vi "UI Tubing Install.vi"(8 "error in":errorcluster) -> (0 "error out":errorcluster)   [LabVIEW 2019, in "Test.lvlib"]
uses:
  Test.lvlib
  Fluidic Process/SubVI/Fluidic Para.ctl
  <vilib>/Utility/file.llb/Read Delimited Spreadsheet (string).vi
  Controller/Controller.lvlib
  Queues/Queues.lvlib
  Fluidic Process/Fluidic Process.lvlib
panel:
  out "Tubing Install":bool
  in  "Stop Process":bool
  out "Remaining Time(s)":dbl
  out "Total Process":string
  out "Current Process":string
  out "Gauge":dbl(knob)=1.2869315802184793e-48 scale=0.0..100.0
  in  "Tubing Install":bool
  in  "Back":bool
  # "/"
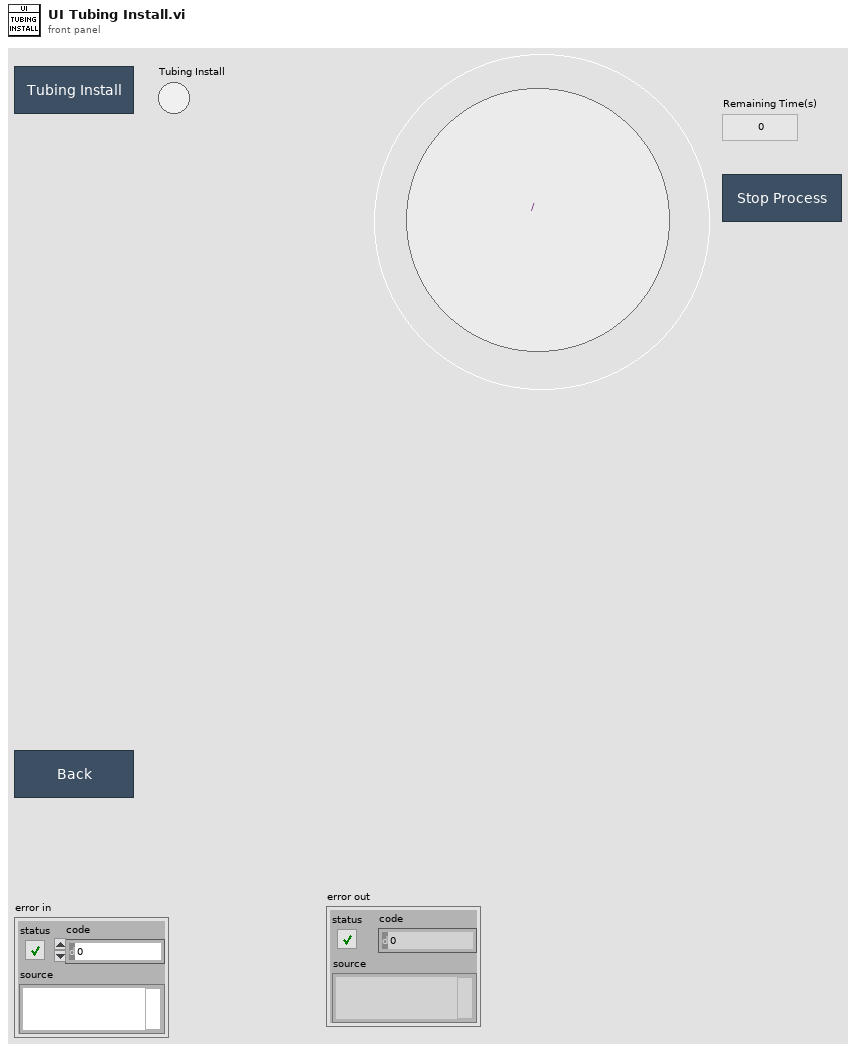
[diagram p1: front panel]
types:
  T1 = enum8{"Enabled", "Disabled", "Disabled and Grayed Out"}
  T2 = typedef "Fluidic Process.lvlib/Fluidic Para.ctl" = cluster{"Read Force Sensor":i32, "Read Regulator":i32, "Read Force Sensor?":bool, "Read Regulator?":bool, "Read Syringe Pump":i32, "Read Syringe Pump?":bool}
  T3 = typedef "Fluidic Process.lvlib/SEQ Data.ctl" = cluster{"Fluidic Process Done?":bool, "Current Process":i32, "Remaining Time":dbl, "Total Process":i32, "Air Sealing":bool, "Force Condition":bool}
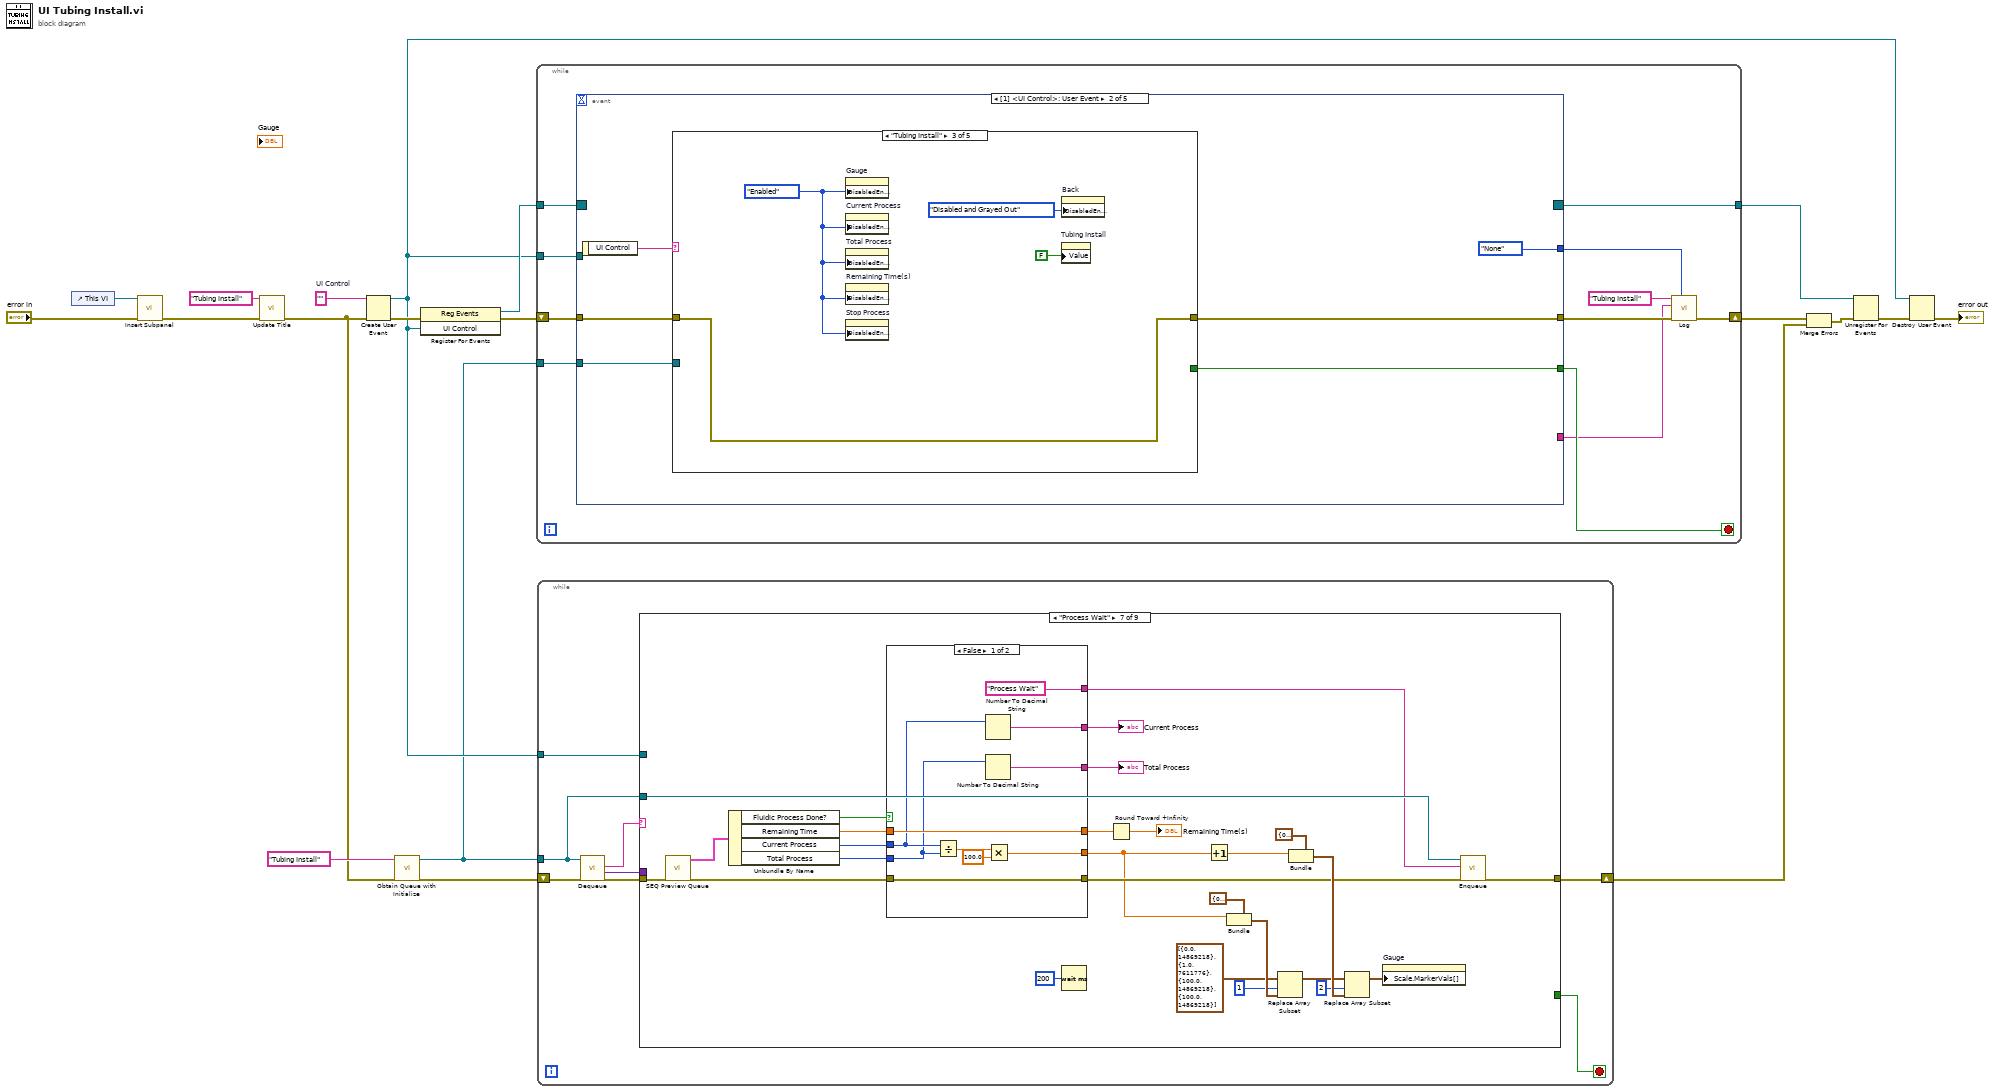
[diagram p0: block diagram]
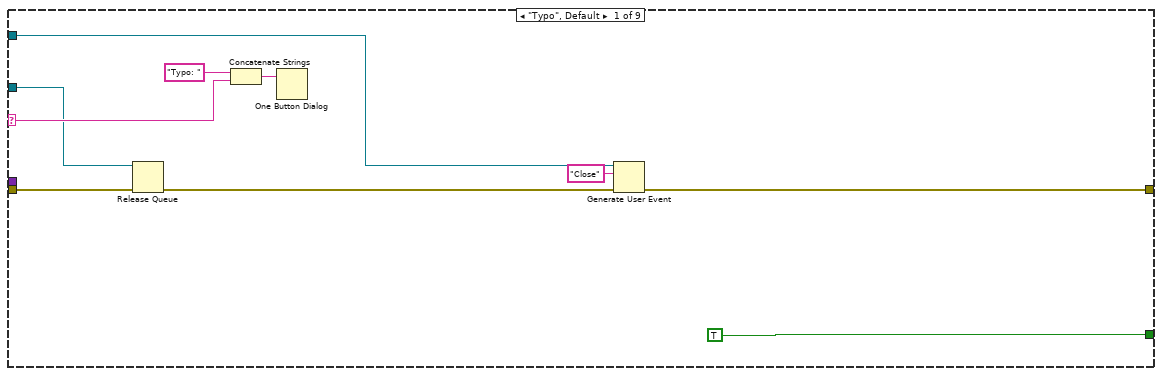
[diagram p2: hidden frame]
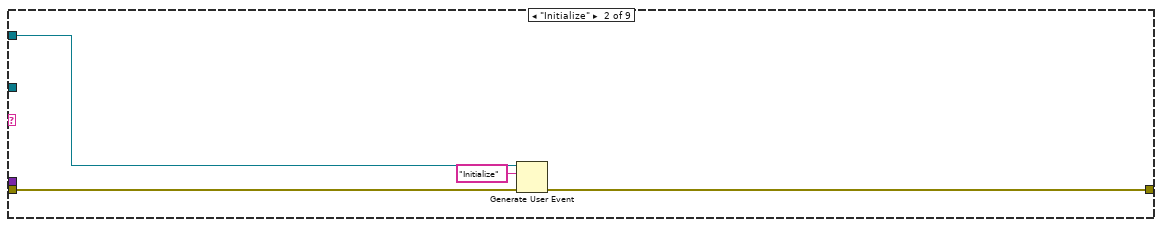
[diagram p3: hidden frame]
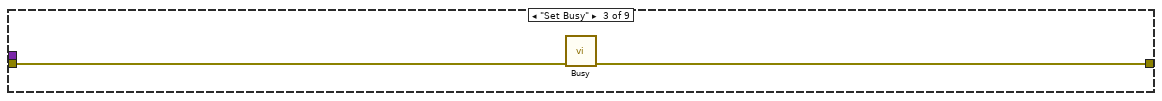
[diagram p4: hidden frame]
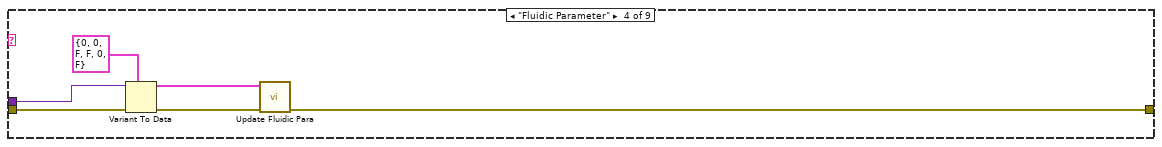
[diagram p5: hidden frame]
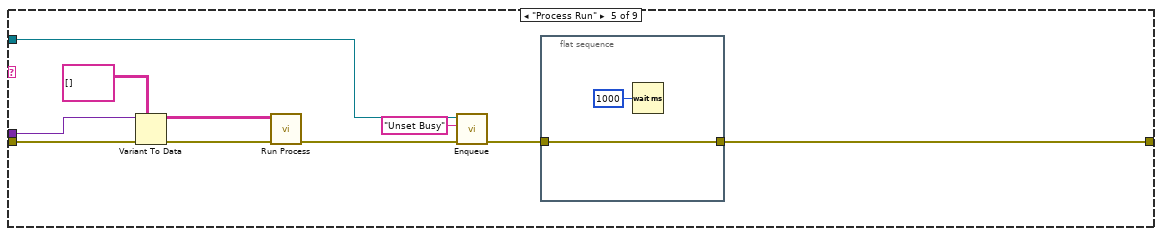
[diagram p6: hidden frame]
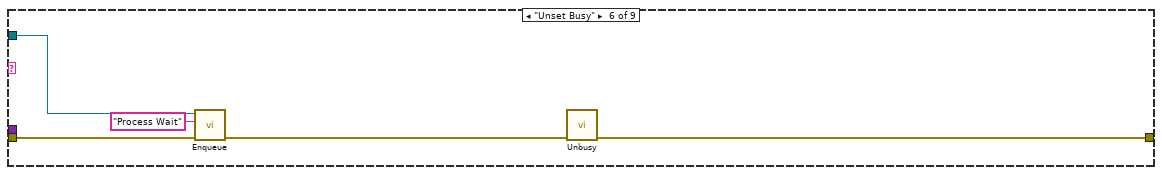
[diagram p7: hidden frame]
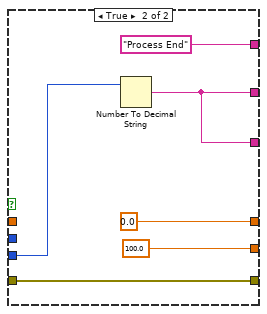
[diagram p8: hidden frame]
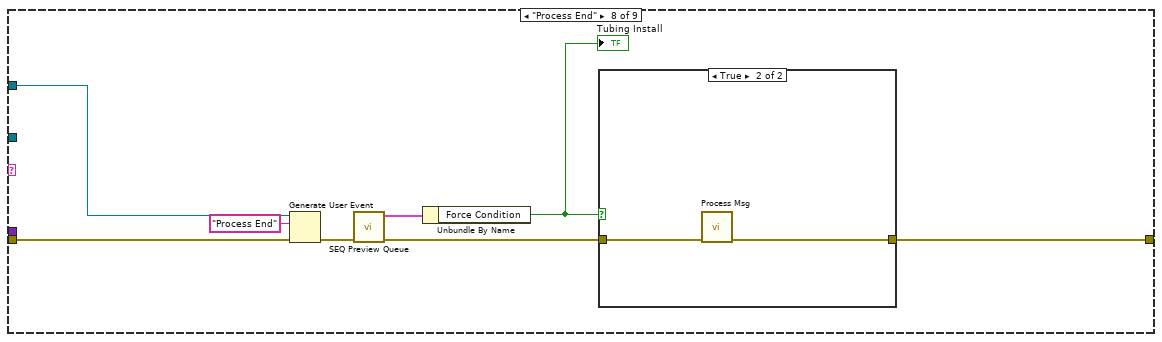
[diagram p9: hidden frame]
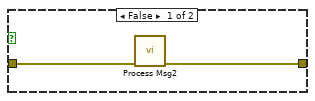
[diagram p10: hidden frame]
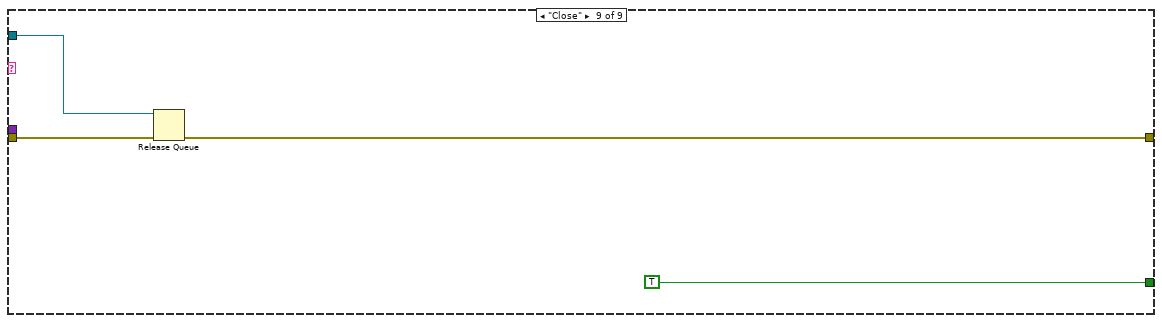
[diagram p11: hidden frame]
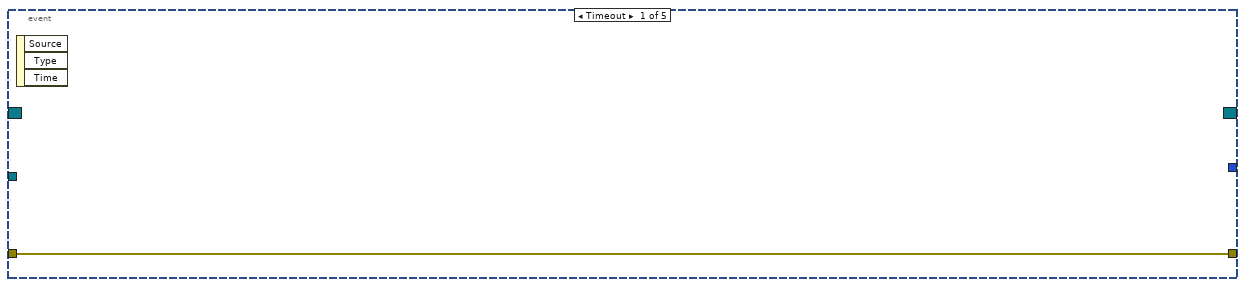
[diagram p12: hidden frame]
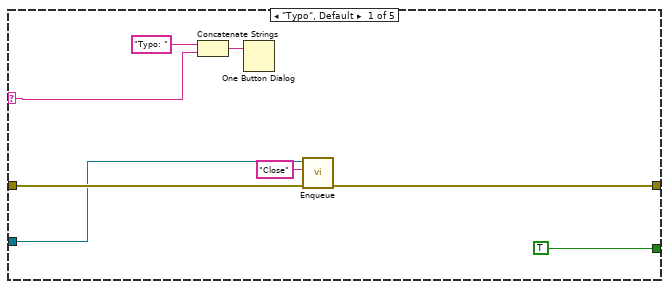
[diagram p13: hidden frame]
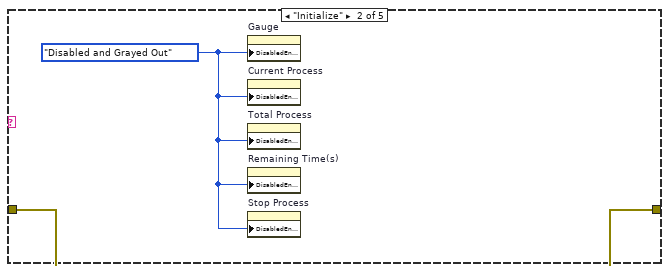
[diagram p14: hidden frame]
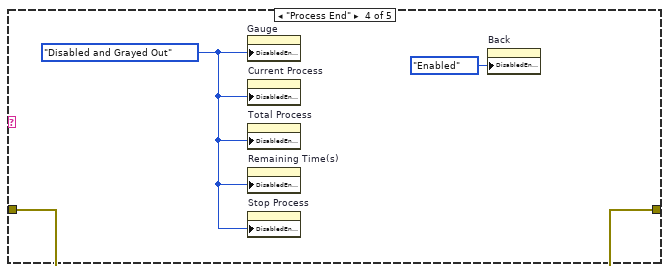
[diagram p15: hidden frame]
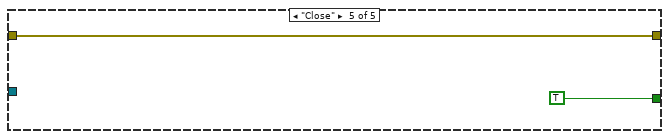
[diagram p16: hidden frame]
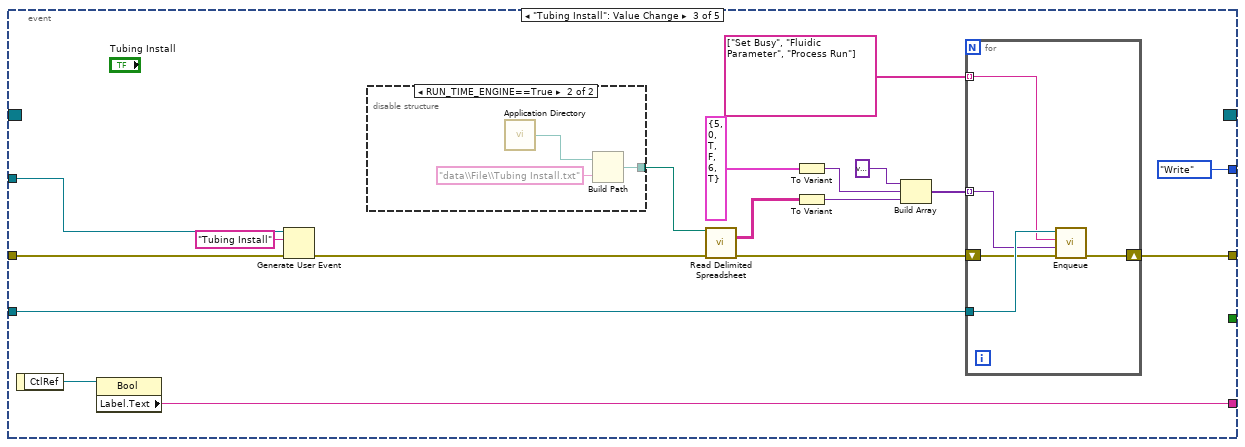
[diagram p17: hidden frame]
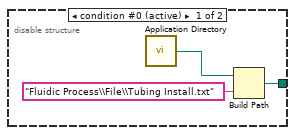
[diagram p18: hidden frame]
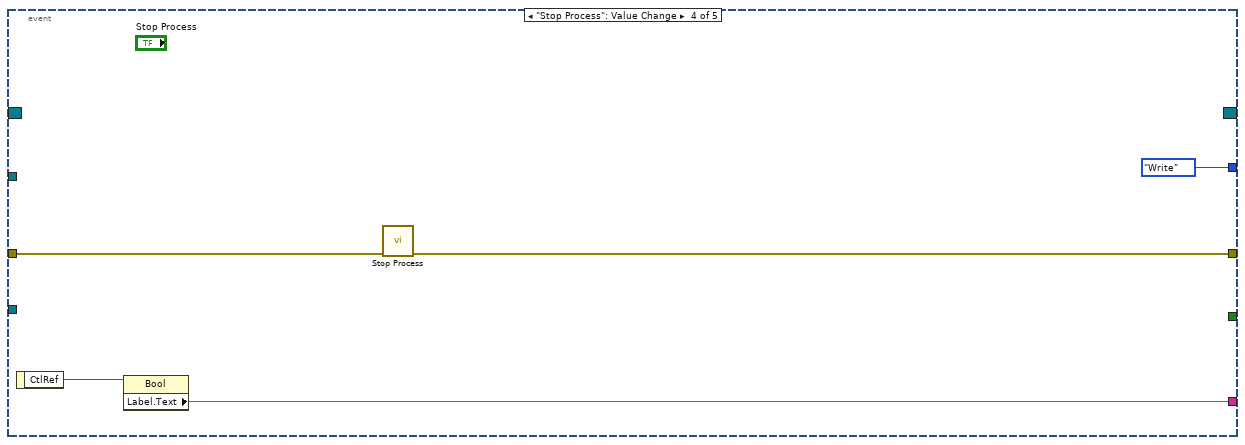
[diagram p19: hidden frame]
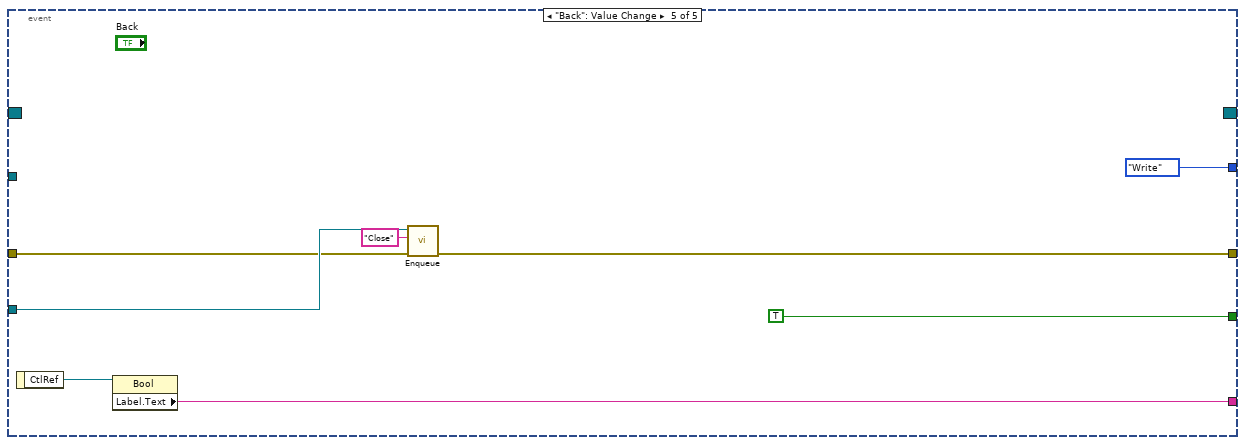
[diagram p20: hidden frame]
diagram:
  w9 = ""  # UI Control
  n1 = control-ref of="This VI"() -> (w8:refnum<vi>)
  n2 = call "Insert Subpanel.vi"("Error In"="error in", "VI Refnum"=w8) -> ("Error Out"=w3:errorcluster)  [unwired: 9 in]
  n3 = call "Update Title.vi"("Error In"=w3, "Title"="Tubing Install") -> ("Error Out"=w2:errorcluster)  [unwired: 9 in]
  n4 = Create User Event(user event datatype=w9, error in=w2) -> (user event=w7:refnum<user-event>, error out=w18:errorcluster)
  n5 = call "Obtain Queue with Initialize.vi"("Error In"=w2, "Queue Name"="Tubing Install") -> ("Error Out"=w6:errorcluster, "Queue out"=w5:refnum<queue>)  [unwired: 8 in]
  n6 = register-events(error in=w18, w7) -> (reference out=w16:refnum<event-registration>, error out=w17:errorcluster)  [unwired: 1 in]
  n7 = while {
    tunnel: w16 -> [w28]
    tunnel: w5 -> [w27]
    shift-right: [w23] -> w14
    shift-left: w17 -> [w30]
    tunnel: [w26] -> w12
    tunnel: w7 -> [w25]
    stop <- w29 stop-if-true
    n8 = event shown="[1] <UI Control>: User Event" {
      selector: w28 -> [_ _ _ _ _]
      dyn-events: [_ _ _ _ _] -> w26
      timeout: _ -> [_ _ _ _ _]
      tunnel: w30 -> [w31 w37 w63 w90 w94]
      tunnel: [_ w33 _ _ TRUE] -> w29
      tunnel: w27 -> [_ w35 w74 _ w96]
      tunnel: [w31 w34 w70 w89 w97] -> w24
      tunnel: w25 -> [_ _ w61 _ _]
      tunnel: [_ enum16{"None", "Write"}."None" ("Action") enum16{"None", "Write"}."Write" ("Action") enum16{"None", "Write"}."Write" ("Action") enum16{"None", "Write"}."Write" ("Action")] -> w21
      tunnel: [_ _ w57 w86 w91] -> w20
      event Timeout {
        n9 = event-data() -> ()  [unwired: 1 in, 3 out]
      }
      event User Event {
        n10 = event-data() -> ("UI Control"=w36:string)  [unwired: 1 in]
        n11 = case shown="\"Tubing Install\"" w36 {
          selector: w36 -> [w40 _ _ _ _]
          tunnel: w37 -> [w45 w47 w51 w54 w56]
          tunnel: w35 -> [w44 _ _ _ _]
          tunnel: [w39 w47 w51 w54 w56] -> w34
          tunnel: [TRUE _ _ _ TRUE] -> w33
          frame "Typo", Default {
            n12 = Concatenate Strings("Typo: " ("string"), w40) -> (w41:string)
            n13 = One Button Dialog(message=w41) -> ()  [unwired: 1 in, 1 out]
            n14 = call "Enqueue.vi"("Error In"=w45, "State"="Close", "Queue in"=w44) -> ("Error Out"=w39:errorcluster)  [unwired: 7 in, 1 out]
          }
          frame "Initialize" {
            w46 = T1."Disabled and Grayed Out" ("Disabled")
            n15 = property on="Gauge" class="Knob (strict)"("DisabledEnum"=w46) -> ()  [unwired: 2 in, 2 out]
            n16 = property on="Current Process" class="Str"("DisabledEnum"=w46) -> ()  [unwired: 2 in, 2 out]
            n17 = property on="Total Process" class="Str"("DisabledEnum"=w46) -> ()  [unwired: 2 in, 2 out]
            n18 = property on="Remaining Time(s)" class="DigNum (strict)"("DisabledEnum"=w46) -> ()  [unwired: 2 in, 2 out]
            n19 = property on="Stop Process" class="Bool"("DisabledEnum"=w46) -> ()  [unwired: 2 in, 2 out]
          }
          frame "Tubing Install" {
            w50 = T1."Enabled" ("Disabled")
            n20 = property on="Gauge" class="Knob (strict)"("DisabledEnum"=w50) -> ()  [unwired: 2 in, 2 out]
            n21 = property on="Current Process" class="Str"("DisabledEnum"=w50) -> ()  [unwired: 2 in, 2 out]
            n22 = property on="Total Process" class="Str"("DisabledEnum"=w50) -> ()  [unwired: 2 in, 2 out]
            n23 = property on="Remaining Time(s)" class="DigNum (strict)"("DisabledEnum"=w50) -> ()  [unwired: 2 in, 2 out]
            n24 = property on="Stop Process" class="Bool"("DisabledEnum"=w50) -> ()  [unwired: 2 in, 2 out]
            n25 = property on="Tubing Install" class="Bool (strict)"("Value"=FALSE ("Tubing Install")) -> ()  [unwired: 2 in, 2 out]
            n26 = property on="Back" class="Bool"("DisabledEnum"=T1."Disabled and Grayed Out" ("Disabled")) -> ()  [unwired: 2 in, 2 out]
          }
          frame "Process End" {
            w53 = T1."Disabled and Grayed Out" ("Disabled")
            n27 = property on="Gauge" class="Knob (strict)"("DisabledEnum"=w53) -> ()  [unwired: 2 in, 2 out]
            n28 = property on="Current Process" class="Str"("DisabledEnum"=w53) -> ()  [unwired: 2 in, 2 out]
            n29 = property on="Total Process" class="Str"("DisabledEnum"=w53) -> ()  [unwired: 2 in, 2 out]
            n30 = property on="Remaining Time(s)" class="DigNum (strict)"("DisabledEnum"=w53) -> ()  [unwired: 2 in, 2 out]
            n31 = property on="Stop Process" class="Bool"("DisabledEnum"=w53) -> ()  [unwired: 2 in, 2 out]
            n32 = property on="Back" class="Bool"("DisabledEnum"=T1."Enabled" ("Disabled")) -> ()  [unwired: 2 in, 2 out]
          }
          frame "Close" {
          }
        }
      }
      event "Tubing Install": Value Change {
        n33 = event-data() -> ("CtlRef"=w58:refnum<vi>)  [unwired: 1 in]
        n34 = property class="Bool"(reference=w58) -> ("Label.Text"=w57:string)  [unwired: 1 in, 2 out]
        n35 = Generate User Event(user event=w61, event data cluster="Tubing Install" ("event data"), error in=w63) -> (error out=w62:errorcluster)  [unwired: 1 in, 1 out]
        n36 = disable-structure shown="RUN_TIME_ENGINE==True" {
          disable-tunnel: [w75 w78] -> w72
          frame condition #0 (active) {
            n37 = call <vilib>:"Application Directory.vi"() -> ("Application Directory"=w77:path)
            n38 = Build Path(base path=w77, name or relative path="Fluidic Process\\File\\Tubing Install.txt") -> (appended path=w75:path)
          }
          frame condition #1 {
            n39 = call <vilib>:"Application Directory.vi"() -> ("Application Directory"=w80:path)
            n40 = Build Path(base path=w80, name or relative path="data\\File\\Tubing Install.txt") -> (appended path=w78:path)
          }
        }
        n41 = call-poly <vilib>:"Read Delimited Spreadsheet.vi"("file path (dialog if empty)"=w72, "error in (no error)"=w62) -> ("all rows"=w71:string[][], "error out"=w73:errorcluster)  [unwired: 8 in, 4 out]
        n42 = To Variant(anything=T2 {"Read Force Sensor"=5, "Read Regulator"=0, "Read Force Sensor?"=TRUE, "Read Regulator?"=FALSE, "Read Syringe Pump"=6, "Read Syringe Pump?"=TRUE} ("Cluster")) -> (Variant=w66:variant)
        n43 = To Variant(anything=w71) -> (Variant=w68:variant)
        n44 = Build Array(variant, w66, w68) -> (w65:variant[])
        n45 = for {
          tunnel: w74 -> [w85]
          shift-right: [w83] -> w70
          shift-left: w73 -> [w84]
          tunnel: string[] ["Set Busy", "Fluidic Parameter", "Process Run"] -> [w82] mode=indexing
          tunnel: w65 -> [w81] mode=indexing
          n46 = call "Enqueue.vi"("Error In"=w84, "Data"=w81, "State"=w82, "Queue in"=w85) -> ("Error Out"=w83:errorcluster)  [unwired: 6 in, 1 out]
        }
      }
      event "Stop Process": Value Change {
        n47 = event-data() -> ("CtlRef"=w87:refnum<vi>)  [unwired: 1 in]
        n48 = property class="Bool"(reference=w87) -> ("Label.Text"=w86:string)  [unwired: 1 in, 2 out]
        n49 = call "Stop Process.vi"("Error In"=w90) -> ("Error Out"=w89:errorcluster)  [unwired: 10 in]
      }
      event "Back": Value Change {
        n50 = event-data() -> ("CtlRef"=w92:refnum<vi>)  [unwired: 1 in]
        n51 = property class="Bool"(reference=w92) -> ("Label.Text"=w91:string)  [unwired: 1 in, 2 out]
        n52 = call "Enqueue.vi"("Error In"=w94, "State"="Close", "Queue in"=w96) -> ("Error Out"=w97:errorcluster)  [unwired: 7 in, 1 out]
      }
    }
    n53 = call "Log.vi"("Action"=w21, "error in"=w24, "State"=w20, "Page Name"="Tubing Install") -> ("error out"=w23:errorcluster)  [unwired: 7 in]
  }
  n54 = while {
    tunnel: w5 -> [w103]
    shift-right: [w101] -> w13
    shift-left: w6 -> [w106]
    tunnel: w7 -> [w100]
    stop <- w99 stop-if-true
    n55 = call "Dequeue.vi"("Error In"=w106, "Queue in"=w103) -> ("Error Out"=w102:errorcluster, "Data"=w104:variant, "State"=w105:string)  [unwired: 6 in, 1 out]
    n56 = case shown="\"Process Wait\"" w105 {
      selector: w105 -> [w114 _ _ _ _ _ _ _ _]
      tunnel: w104 -> [_ _ _ w127 w137 _ _ _ _]
      tunnel: w103 -> [w107 _ _ _ w132 w144 w150 _ w202]
      tunnel: w102 -> [w109 w120 w122 w128 w138 w145 w172 w196 w204]
      tunnel: [TRUE _ _ _ _ _ _ _ TRUE] -> w99
      tunnel: [w112 w119 w121 w123 w129 w141 w156 w190 w203] -> w101
      tunnel: w100 -> [w111 w118 _ _ _ _ _ w195 _]
      frame "Typo", Default {
        n57 = Release Queue(queue=w107, error in (no error)=w109) -> (error out=w108:errorcluster)  [unwired: 1 in, 2 out]
        n58 = Concatenate Strings("Typo: " ("string"), w114) -> (w116:string)
        n59 = One Button Dialog(message=w116) -> ()  [unwired: 1 in, 1 out]
        n60 = Generate User Event(user event=w111, event data cluster="Close" ("event data"), error in=w108) -> (error out=w112:errorcluster)  [unwired: 1 in, 1 out]
      }
      frame "Initialize" {
        n61 = Generate User Event(user event=w118, event data cluster="Initialize" ("event data"), error in=w120) -> (error out=w119:errorcluster)  [unwired: 1 in, 1 out]
      }
      frame "Set Busy" {
        n62 = call "Busy.vi"("Error In"=w122) -> ("Error Out"=w121:errorcluster)  [unwired: 10 in]
      }
      frame "Fluidic Parameter" {
        n63 = Variant To Data(error in=w128, type=T2 {"Read Force Sensor"=0, "Read Regulator"=0, "Read Force Sensor?"=FALSE, "Read Regulator?"=FALSE, "Read Syringe Pump"=0, "Read Syringe Pump?"=FALSE} ("Cluster"), Variant=w127) -> (data=w124:T2, error out=w125:errorcluster)
        n64 = call "Update Fluidic Para.vi"("Error In"=w125, "Fluidic Para"=w124) -> ("Error Out"=w123:errorcluster)  [unwired: 9 in]
      }
      frame "Process Run" {
        n65 = Variant To Data(error in=w138, type=string[][] [] ("all rows"), Variant=w137) -> (data=w134:string[][], error out=w135:errorcluster)
        n66 = call "Run Process.vi"("Error In"=w135, "Fluidic Process in"=w134) -> ("Error Out"=w133:errorcluster)  [unwired: 9 in]
        n67 = call "Enqueue.vi"("Error In"=w133, "State"="Unset Busy", "Queue in"=w132) -> ("Error Out"=w130:errorcluster)  [unwired: 7 in, 1 out]
        n68 = flat-sequence {
          tunnel: w130 -> [w140]
          tunnel: [w140] -> w129
          frame #0 {
            n69 = Wait (ms)(milliseconds to wait=u32 1000) -> ()  [unwired: 1 out]
          }
        }
      }
      frame "Unset Busy" {
        n70 = call "Enqueue.vi"("Error In"=w145, "State"="Process Wait", "Queue in"=w144) -> ("Error Out"=w142:errorcluster)  [unwired: 7 in, 1 out]
        n71 = call "Unbusy.vi"("Error In"=w142) -> ("Error Out"=w141:errorcluster)  [unwired: 10 in]
      }
      frame "Process Wait" {
        n72 = call "SEQ Preview Queue.vi"("error in"=w172) -> ("error out"=w169:errorcluster, "SEQ Data"=w171:T3)  [unwired: 9 in]
        n73 = Unbundle By Name(w171) -> ("Fluidic Process Done?"=w170:bool, "Remaining Time"=w155:dbl, "Current Process"=w154:i32, "Total Process"=w153:i32)
        n74 = case shown="False" w170 {
          tunnel: w169 -> [w180 w188]
          tunnel: [w180 w188] -> w157
          tunnel: w155 -> [w179 _]
          tunnel: w154 -> [w177 _]
          tunnel: w153 -> [w176 w187]
          tunnel: [w179 0.0 ("Remaining Time")] -> w151
          tunnel: [w178 100.0] -> w152
          tunnel: [w175 w186] -> w149
          tunnel: [w174 w186] -> w148
          tunnel: ["Process Wait" "Process End"] -> w147
          frame False {
            n75 = Divide(x=w177, y=w176) -> (x/y=w182:dbl)
            n76 = Number To Decimal String(number=w177) -> (decimal integer string=w175:string)  [unwired: 1 in]
            n77 = Number To Decimal String(number=w176) -> (decimal integer string=w174:string)  [unwired: 1 in]
            n78 = Multiply(x=w182, y=100.0) -> (x*y=w178:dbl)
          }
          frame True {
            n79 = Number To Decimal String(number=w187) -> (decimal integer string=w186:string)  [unwired: 1 in]
          }
        }
        "Total Process" <- w148
        "Current Process" <- w149
        n80 = Wait (ms)(milliseconds to wait=u32 200) -> ()  [unwired: 1 out]
        n81 = Round Toward +Infinity(x=w151) -> (ceil(x): smallest int >= x=→"Remaining Time(s)":dbl)
        n82 = Increment(x=w152) -> (x+1=w165:dbl)
        n83 = Bundle(cluster=cluster{dbl, i32} {0.0, 7611776}, w152) -> (w164:cluster{dbl, i32})  [unwired: 1 in]
        n84 = Replace Array Subset(array=cluster{dbl, u32}[] [{0.0, 14869218}, {1.0, 7611776}, {100.0, 14869218}, {100.0, 14869218}] ("Scale.Marker Values[]"), new element=w164, index=1) -> (w166:cluster{dbl, u32}[])
        n85 = Bundle(cluster=cluster{dbl, i32} {0.0, 14869218}, w165) -> (w167:cluster{dbl, i32})  [unwired: 1 in]
        n86 = Replace Array Subset(array=w166, new element=w167, index=2) -> (w168:cluster{dbl, u32}[])
        n87 = property on="Gauge" class="Knob (strict)"("Scale.MarkerVals[]"=w168) -> ()  [unwired: 2 in, 2 out]
        n88 = call "Enqueue.vi"("Error In"=w157, "State"=w147, "Queue in"=w150) -> ("Error Out"=w156:errorcluster)  [unwired: 7 in, 1 out]
      }
      frame "Process End" {
        n89 = Generate User Event(user event=w195, event data cluster="Process End" ("event data"), error in=w196) -> (error out=w193:errorcluster)  [unwired: 1 in, 1 out]
        n90 = call "SEQ Preview Queue.vi"("error in"=w193) -> ("error out"=w191:errorcluster, "SEQ Data"=w192:T3)  [unwired: 9 in]
        n91 = Unbundle By Name(w192) -> ("Force Condition"=w189:bool)
        "Tubing Install" <- w189
        n92 = case shown="True" w189 {
          tunnel: w191 -> [w198 w200]
          tunnel: [w197 w199] -> w190
          frame False {
            n93 = call "Process Msg2"("error in (no error)"=w198) -> ("error out"=w197:errorcluster)  [unwired: 9 in, 1 out]
          }
          frame True {
            n94 = call "Process Msg"("error in (no error)"=w200) -> ("error out"=w199:errorcluster)  [unwired: 9 in, 1 out]
          }
        }
      }
      frame "Close" {
        n95 = Release Queue(queue=w202, error in (no error)=w204) -> (error out=w203:errorcluster)  [unwired: 1 in, 2 out]
      }
    }
  }
  n96 = Merge Errors(w14, w13) -> (w11:errorcluster)
  n97 = Unregister For Events(event registration refnum=w12, error in=w11) -> (error out=w10:errorcluster)
  n98 = Destroy User Event(user event=w7, error in=w10) -> (error out=→"error out":errorcluster)
